vi "Global - UI Stream and Variable Connections.vi"() -> ()   [LabVIEW 2018]
uses:
  Support/Message Queue/Message Cluster.ctl
  Support/Message Queue/Message.ctl
  Controls/VTF Sensors.ctl
  support/Message Queue/Message Queue.lvlib
panel:
  in  "Variable References":T1={"CPU Usage"="ni.var.psp://192.168.91.21/Shared Variables/CPU Usage", "Contiguous Memory"="ni.var.psp://192.168.91.21/Shared Variables/Contiguous Memory", "VTF Sensors"=""}
  in  "RT Message Stream":refnum<k21>
  in  "UI Command Stream":refnum<k21>
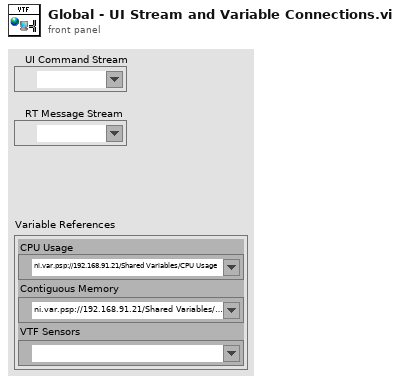
[diagram p1: front panel]
types:
  T1 = cluster{"CPU Usage":refnum<k21>, "Contiguous Memory":refnum<k21>, "VTF Sensors":refnum<k21>}
diagram:
